vi "acquire.vi"(8 "error in (no error)":errorcluster, 11 "Resonance Curve in":refnum<class "Resonance Curve.lvclass">) -> (0 "error out":errorcluster, 3 "Resonance Curve out":refnum<class "Resonance Curve.lvclass">)   [LabVIEW 2020, in "Resonance Curve.lvclass"]
uses:
  Resonance Curve.lvclass
  Resonance Curve Data/Resonance Curve Data.lvclass
  Resonance Curve.lvclass/Resonance Curve.ctl
  Function Generator/Function Generator.lvclass
  Lock-In Amplifier/Lock-In Amplifier.lvclass
panel:
  out "Resonance Curve Data out":refnum<class "Resonance Curve Data.lvclass">
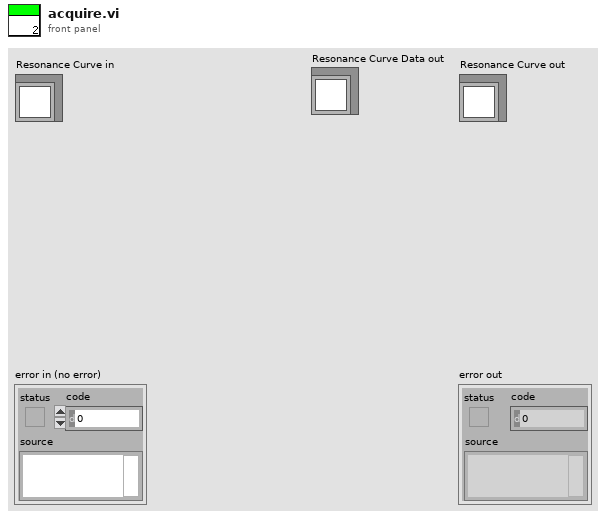
[diagram p1: front panel]
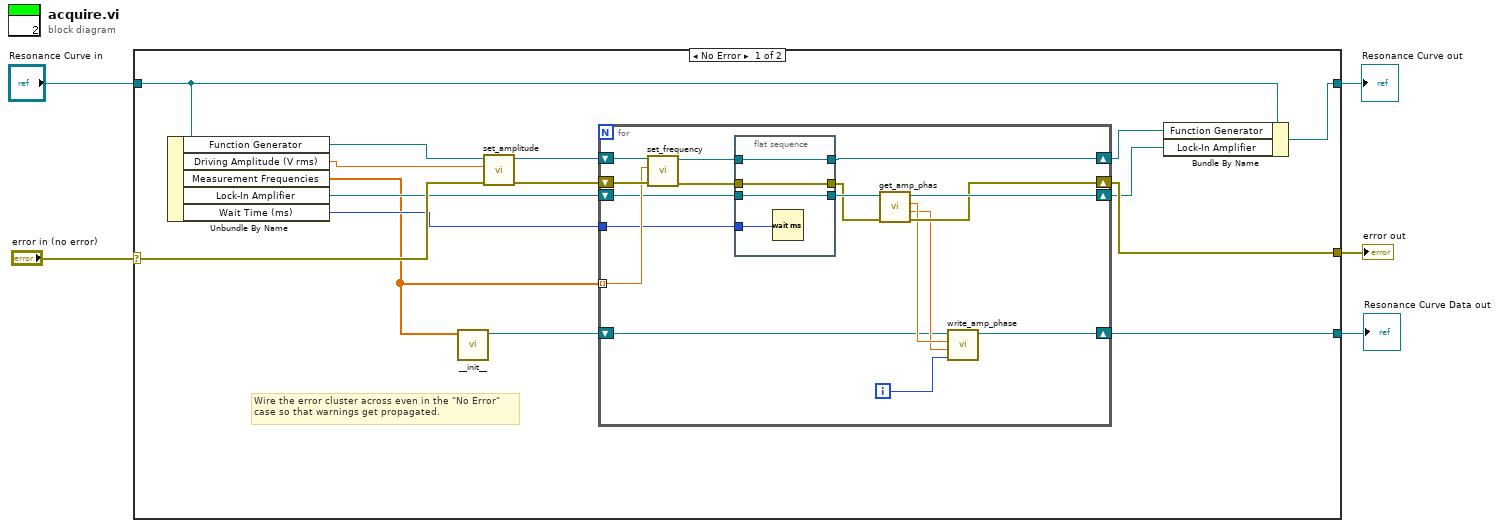
[diagram p0: block diagram]
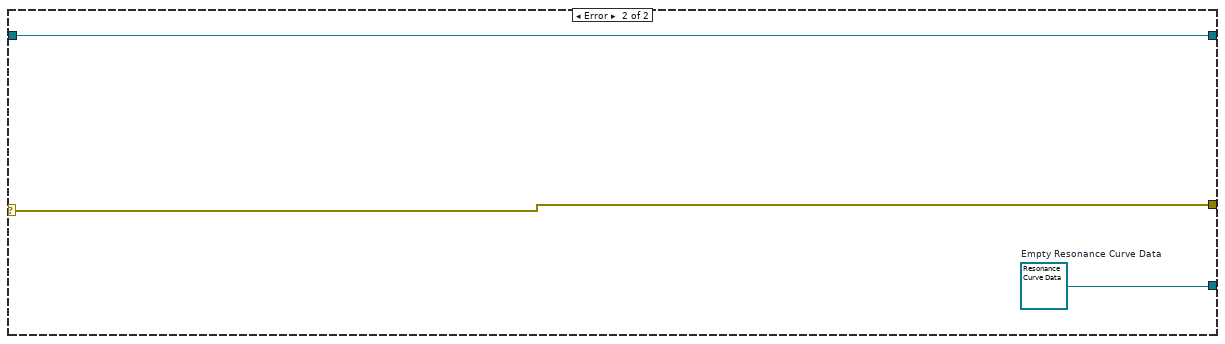
[diagram p2: hidden frame]
diagram:
  n1 = case shown="No Error" "error in (no error)" {
    selector: "error in (no error)" -> [w18 w44]
    tunnel: [w13 w44] -> w4
    tunnel: [w9 w43] -> w2
    tunnel: "Resonance Curve in" -> [w12 w43]
    tunnel: [w6 w42] -> w1
    frame No Error {
      # "Wire the error cluster across even in the \"No Error\"\ncase so that warnings get propagated."
      n2 = Unbundle By Name(w12) -> ("Function Generator"=w20:refnum<class "Function Generator.lvclass">, "Driving Amplitude (V rms)"=w19:dbl, "Measurement Frequencies"=w8:dbl[], "Lock-In Amplifier"=w17:refnum<class "Lock-In Amplifier.lvclass">, "Wait Time (ms)"=w14:u32)
      n3 = call "__init__.vi"("Frequencies"=w8) -> ("Resonance Curve Data out"=w7:refnum<class "Resonance Curve Data.lvclass">)  [unwired: 9 in, 1 out]
      n4 = call-dynamic "set_amplitude.vi"("error in (no error)"=w18, "Amplitude"=w19, "Function Generator in"=w20) -> ("error out"=w15:errorcluster, "Function Generator out"=w16:refnum<class "Function Generator.lvclass">)  [unwired: 7 in]
      n5 = for {
        tunnel: w8 -> [w35] mode=indexing
        shift-right: [w28] -> w11
        shift-left: w16 -> [w37]
        shift-right: [w26] -> w13
        shift-left: w15 -> [w36]
        shift-right: [w27] -> w10
        shift-left: w17 -> [w31]
        tunnel: w14 -> [w32]
        shift-right: [w23] -> w6
        shift-left: w7 -> [w21]
        i -> [w22]
        n6 = call-dynamic "set_frequency.vi"("error in (no error)"=w36, "Frequency"=w35, "Function Generator in"=w37) -> ("error out"=w33:errorcluster, "Function Generator out"=w34:refnum<class "Function Generator.lvclass">)  [unwired: 7 in]
        n7 = flat-sequence {
          tunnel: w34 -> [w39]
          tunnel: w33 -> [w40]
          tunnel: w32 -> [w41]
          tunnel: [w40] -> w29
          tunnel: [w39] -> w28
          tunnel: w31 -> [w38]
          tunnel: [w38] -> w30
          frame #0 {
            n8 = Wait (ms)(milliseconds to wait=w41) -> ()  [unwired: 1 out]
          }
        }
        n9 = call-dynamic "get_amp_phas.vi"("error in (no error)"=w29, "Lock-In Amplifier in"=w30) -> ("error out"=w26:errorcluster, "Phase (rad)"=w24:dbl, "Amplitude (V rms)"=w25:dbl, "Lock-In Amplifier out"=w27:refnum<class "Lock-In Amplifier.lvclass">)  [unwired: 6 in]
        n10 = call "write_amp_phase.vi"("Index"=w22, "Phase (rad)"=w24, "Amplitude (V)"=w25, "Resonance Curve Data in"=w21) -> ("Resonance Curve Data out"=w23:refnum<class "Resonance Curve Data.lvclass">)  [unwired: 7 in]
      }
      n11 = Bundle By Name(cluster=w12, "Function Generator"=w11, "Lock-In Amplifier"=w10) -> (w9:refnum<class "Resonance Curve.lvclass">)
    }
    frame Error {
      w42 = refnum<class "Resonance Curve Data.lvclass"> refnum  # Empty Resonance Curve Data
    }
  }
  "error out" <- w4
  "Resonance Curve out" <- w2
  "Resonance Curve Data out" <- w1
